vi "merge_Totalize.vi"   [LabVIEW 2020, in "NI_FunctionBlockMergeVIs.lvlib"]
doc: "Calculates a trapezoidal Riemann sum to approximate the integral of <B>input</B>."
uses:
  <vilib>/functionblocks/NI_FunctionBlockMergeVIs.lvlib
  <vilib>/functionblocks/Accumulate/Totalize/Totalize.ctl
  <vilib>/functionblocks/FB Core/FB Core.xnode
  <vilib>/functionblocks/NI_FunctionBlock Libraries.lvlib
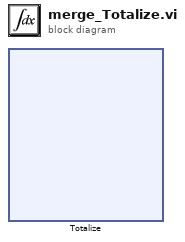
[diagram p0: block diagram]
diagram:
  n1 = xnode "Totalize"() -> ()  [unwired: 6 in, 2 out]
